vi "K6514_SimpleVoltageReader.vi"() -> ()   [LabVIEW 2024]
panel:
  in  "Range":dbl(ring)=200.0 items=["200 V"=200.0, "20 V"=20.0, "2 V"=2.0]
  out "Waveform Graph":dbl[](graph)
  in  "file path (use dialog)":path
  in  "stop":bool
  out "error out":errorcluster
  out "Voltage (V)":dbl
  in  "VISA resource name":refnum<visa-resource-name>
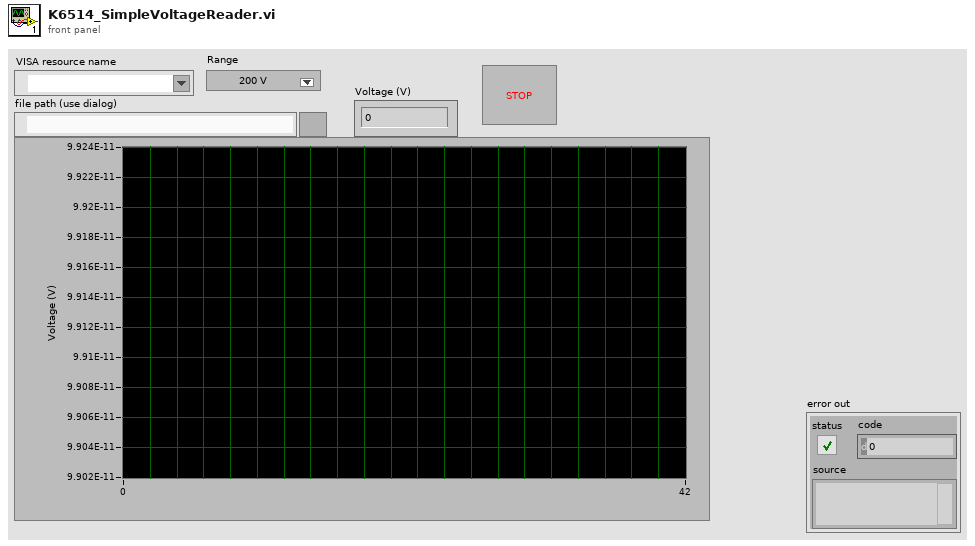
[diagram p1: front panel]
types:
  T1 = enum16{"open", "replace", "create", "open or create", "replace or create", "replace or create with confirmation"}
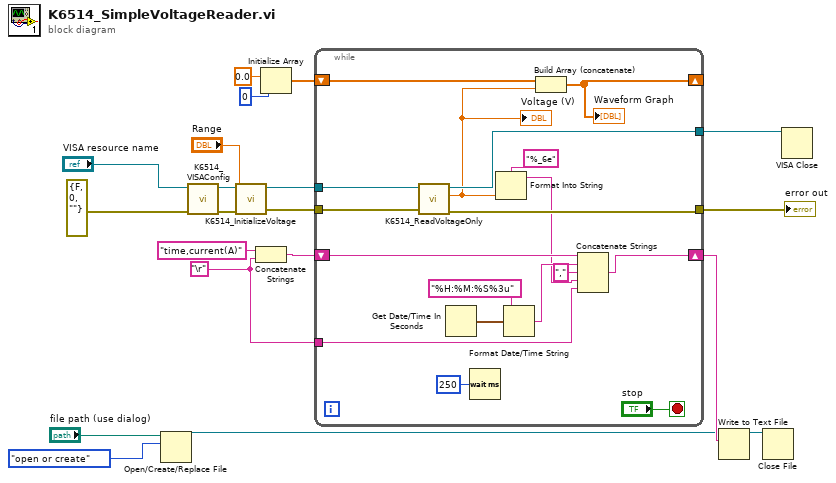
[diagram p0: block diagram]
diagram:
  w14 = "\r"
  n1 = Open/Create/Replace File(file path (use dialog)="file path (use dialog)", operation (0:open)=T1."open or create") -> (refnum out=w9:refnum<file>)  [unwired: 4 in, 2 out]
  n2 = call "K6514_VISAConfig.vi"("error in (no error)"=errorcluster {"status"=FALSE, "code"=0, "source"=""}, "VISA resource name"="VISA resource name") -> ("error out"=w8:errorcluster, "reference out"=w7:refnum<visa-resource-name>)  [unwired: 8 in]
  n3 = call "K6514_InitializeVoltage.vi"("error in (no error)"=w8, "Range"="Range", "VISA resource name"=w7) -> ("error out"=w19:errorcluster, "VISA resource name out"=w20:refnum<visa-resource-name>)  [unwired: 7 in]
  n4 = Concatenate Strings("time,current(A)" ("string"), w14) -> (w16:string)
  n5 = Initialize Array(0.0 ("element"), 0 ("dimension size")) -> (w2:dbl[])
  n6 = while {
    tunnel: w20 -> [w38]
    tunnel: [w35] -> w17
    tunnel: w19 -> [w37]
    tunnel: [w36] -> w18
    shift-right: [w30] -> w10
    shift-left: w16 -> [w31]
    tunnel: w14 -> [w29]
    shift-right: [w22] -> _
    shift-left: w2 -> [w23]
    stop <- "stop" stop-if-true
    n7 = call "K6514_ReadVoltageOnly.vi"("error in (no error)"=w37, "VISA resource name"=w38) -> ("error out"=w36:errorcluster, "Voltage(V)"=w21:dbl, "VISA resource name out"=w35:refnum<visa-resource-name>)  [unwired: 5 in, 1 out]
    "Voltage (V)" <- w21
    n8 = Get Date/Time In Seconds() -> (seconds since 1Jan1904=w34:timestamp)
    n9 = Wait (ms)(milliseconds to wait=u32 250) -> ()  [unwired: 1 out]
    n10 = Format Into String(format string="%_6e", w21) -> (resulting string=w26:string)  [unwired: 2 in, 1 out]
    n11 = Format Date/Time String(time format string (%c)="%H:%M:%S%3u", seconds (now)=w34) -> (date/time string=w32:string)  [unwired: 1 in]
    n12 = Build Array (concatenate)(w23, w21) -> (w22:dbl[])
    "Waveform Graph" <- w22
    n13 = Concatenate Strings(w31, w32, "," ("string"), w26, w29) -> (w30:string)
  }
  "error out" <- w18
  n14 = Write to Text File(file (use dialog)=w9, text=w10) -> (refnum out=w11:refnum<file>)  [unwired: 2 in, 2 out]
  n15 = Close File(refnum=w11) -> ()  [unwired: 1 in, 2 out]
  n16 = VISA Close(VISA resource name=w17) -> ()  [unwired: 1 in, 1 out]
